vi "run.update_free.vi"(8 "error in":errorcluster, 11 "RunUpdateStaging in":refnum<class "RunUpdateStaging.lvclass">) -> (0 "error out":errorcluster, 3 "RunUpdateStaging out":refnum<class "RunUpdateStaging.lvclass">)   [LabVIEW 2020, in "RunUpdateStaging.lvclass"]
doc: "Releases the handle and its associated resources."
uses:
  RunUpdateStaging.lvclass
  RunUpdateStaging.lvclass/RunUpdateStaging.ctl
  client.lvlib
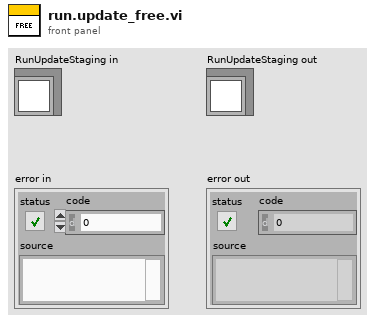
[diagram p1: front panel]
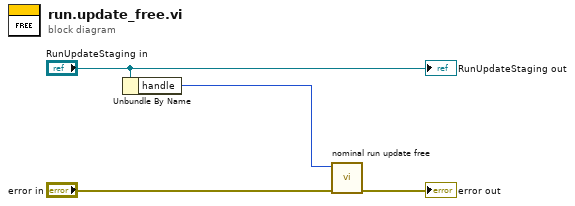
[diagram p0: block diagram]
diagram:
  n1 = Unbundle By Name("RunUpdateStaging in") -> ("handle"=w2:i32)
  n2 = call "nominal run update free.vi"("error in (no error)"="error in", "staging"=w2) -> ("error out"=→"error out":errorcluster)  [unwired: 8 in, 1 out]
  "RunUpdateStaging out" <- "RunUpdateStaging in"
